vi "Read Buffered Error.vi"(8 "error in":errorcluster, 9 "timeout in ms (0)":i32, 11 "Standard Engine Runtime in":refnum<class "synchronous engine runtime.lvclass">) -> (0 "error out":errorcluster, 2 "Engine Error":errorcluster, 3 "Standard Engine Runtime out":refnum<class "synchronous engine runtime.lvclass">)   [LabVIEW 2013, in "synchronous engine runtime.lvclass"]
uses:
  synchronous engine runtime.lvclass
  synchronous engine runtime.lvclass/synchronous engine runtime.ctl
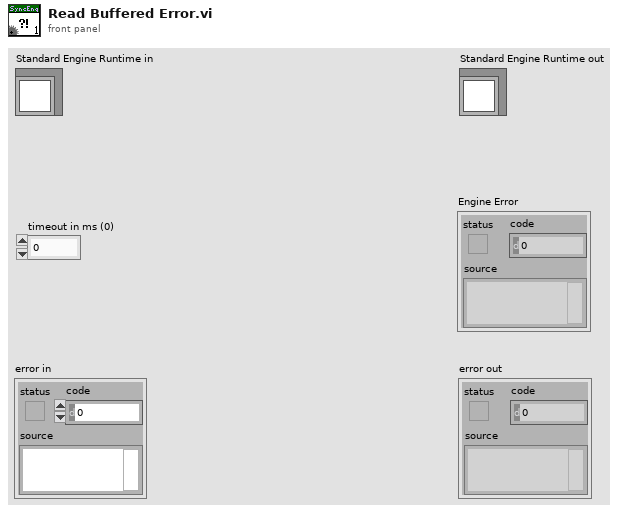
[diagram p1: front panel]
types:
  T1 = typedef "synchronous engine runtime.lvclass/notifier.ctl" = cluster{"Engine State":T2, "error constant":errorcluster}
  T2 = typedef "Engine Runtime Interface.lvclass/Execution States.ctl" = enum16{"Initializing", "Paused (Initialized)", "Running", "Set Safe Outputs", "Uninitializing", "Stopped (Uninitialized)", "Error (Uninitialized)", "Safe State (Uninitialized)", "Closed"}
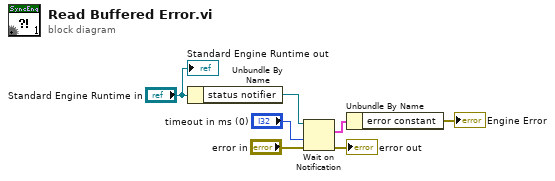
[diagram p0: block diagram]
diagram:
  n1 = Unbundle By Name("Standard Engine Runtime in") -> ("status notifier"=w6:refnum<notifier>)
  n2 = Wait on Notification(notifier=w6, timeout in ms (-1)="timeout in ms (0)", error in (no error)="error in") -> (notification=w2:T1, error out=→"error out":errorcluster)  [unwired: 1 in, 2 out]
  n3 = Unbundle By Name(w2) -> ("error constant"=→"Engine Error":errorcluster)
  "Standard Engine Runtime out" <- "Standard Engine Runtime in"
